vi "Dashboard Main_1920_1080.vi"() -> ()   [LabVIEW 2020]
uses:
  <vilib>/Rock Robotics/WPI/ThirdParty/JAS_Junk/TrajLib/TypeDef/FieldDisp_ElementPicture.ctl
  <vilib>/event_ctls.llb/eventvkey.ctl
  <vilib>/Rock Robotics/WPI/ThirdParty/JAS_Junk/TrajLib/Rotation2d_CreateAngle.vi
  <vilib>/Rock Robotics/WPI/ThirdParty/JAS_Junk/TrajLib/Translation2d_Create.vi
  <vilib>/Rock Robotics/WPI/ThirdParty/JAS_Junk/TrajLib/VI/FieldDisp_Element_Rotate.vi
  <vilib>/Rock Robotics/WPI/ThirdParty/JAS_Junk/TrajLib/Conv_Meters_Inches.vi
  <vilib>/Rock Robotics/WPI/ThirdParty/JAS_Junk/TrajLib/Conv_Radians_Deg.vi
  <vilib>/Rock Robotics/WPI/Dashboard/WPI_DashboardLogging Global.vi
  <vilib>/Rock Robotics/Network Tables/NT Read Numeric Array.vi
  <vilib>/picture/pixmap.llb/Flatten Pixmap.vi
  <vilib>/picture/pictutil.llb/Create Mask.vi
  <vilib>/picture/picture.llb/Draw Flattened Pixmap.vi
  <vilib>/Rock Robotics/WPI/ThirdParty/JAS_Junk/TrajLib/Trajectory_Library.lvlib
panel:
  out "Camera Perf":string
  in  "Camera Settings":T1={"Frame Rate"=30, "Compression"=30, "Size"=1, "DB Camera Config"=FALSE} {"Frame Rate" scale=1.0..30.0; "Compression" scale=100.0..-1.0; "Size" items=["640x480", "320x240", "160x120"]}
  in  "TCP":refnum<k5>
  in  "Rec Mode":enum32{"Stop", "Record", "Playback"}(radio)
  out "Robot IP":string
  out "Image Message":string="Timeout in Camera Communications"
  in  "Dashboard Tab":T2(tab)
  in  "Select Auto":string(combo)="Select Autonomous ..."
  out "NT Connection":bool
  out "MotorChart R":cluster{"Numeric":dbl, "Numeric":dbl}(graph)
  out "MotorChart L":cluster{"Numeric":dbl, "Numeric":dbl}(graph)
  out "MotorSliders R":cluster{"MotorSlide1":dbl, "MotorSlide2":dbl} {"MotorSlide2" scale=-1.0..1.0 scale format="%#_2e"; "MotorSlide1" scale=-1.0..1.0 scale format="%#_2e"}
  out "MotorSliders L":cluster{"MotorSlide1":dbl, "MotorSlide2":dbl} {"MotorSlide2" scale=-1.0..1.0 scale format="%#_2e"; "MotorSlide1" scale=-1.0..1.0 scale format="%#_2e"}
  out "Gyro":dbl(knob) scale=0.0..360.0
  out "JS1 Z":dbl(slide) scale=-1.0..1.0 scale format="%#_2e"
  out "JS1 Graph":cluster{"X":dbl, "Y":dbl}[](graph)
  out "JS1 Buttons":T3
  out "JS2 Z":dbl(slide) scale=-1.0..1.0 scale format="%#_2e"
  out "JS2 Graph":cluster{"X":dbl, "Y":dbl}[](graph)
  out "JS2 Buttons":T3
  out "Mode":T4(ring)=enum."Auto Disabled"
  out "Right Camera Perf":cluster{"Bandwidth (Mbps)":dbl, "FPS":dbl}
  in  "DB/String 9":string
  in  "DB/String 8":string
  in  "DB/String 7":string
  in  "DB/String 6":string
  in  "DB/String 5":string
  in  "DB/String 4":string
  in  "DB/String 3":string
  in  "DB/String 2":string
  in  "DB/String 1":string
  in  "DB/String 0":string
  in  "DB/Slider 0":dbl(slide) scale=0.0..5.0
  in  "DB/Slider 1":dbl(slide) scale=0.0..5.0
  in  "DB/Slider 2":dbl(slide) scale=0.0..5.0
  in  "DB/Slider 3":dbl(slide) scale=0.0..5.0
  out "DB/LED 3":bool
  out "DB/LED 2":bool
  out "DB/LED 1":bool
  out "DB/LED 0":bool
  in  "DB/Button 3":bool
  in  "DB/Button 2":bool
  in  "DB/Button 1":bool
  in  "DB/Button 0":bool caption="New Name"
  out "ROBOT":T5
  out "Field Picture":picture
  in  "Test Slider":dbl(slide) scale=0.0..100.0 scale format="%#_3g"
  in  "On/Off":bool caption="Solenoid"
  in  "Test Name":u16(ring) items=["Select the test to run..."]
  in  "Test Tree":string(tree)
  in  "Motor":cluster{"Value":dbl, "Enable":bool} {"Value" scale=-1.0..1.0 scale format="%#_3g"}
  out "Progress":T6 {"Test Progress" scale=0.0..100.0}
  in  "Rev/Fwd":cluster{"Forward":bool, "Reverse":bool}
  in  "Test Ring":u16(ring) items=["Monochrome", "Color"]
  in  "CheckList":i32(listbox)
  out "Tree":string(tree)
  out "Camera Image":T7(plugin-control)
  out "Background":bool
  in  "Camera Name":string(combo)="No Camera Selection"
  # "HW"
  # "Joysticks"
  # "Drive Motors"
  # "Front"
  # "Right"
  # "Left"
  # "Back"
  # "This tab is a great place for autonomous settings and robot-specific values.\nPlace controls and indicators inside this tab and match name to\nDashboard Variables on robot. You can also delete this comment."
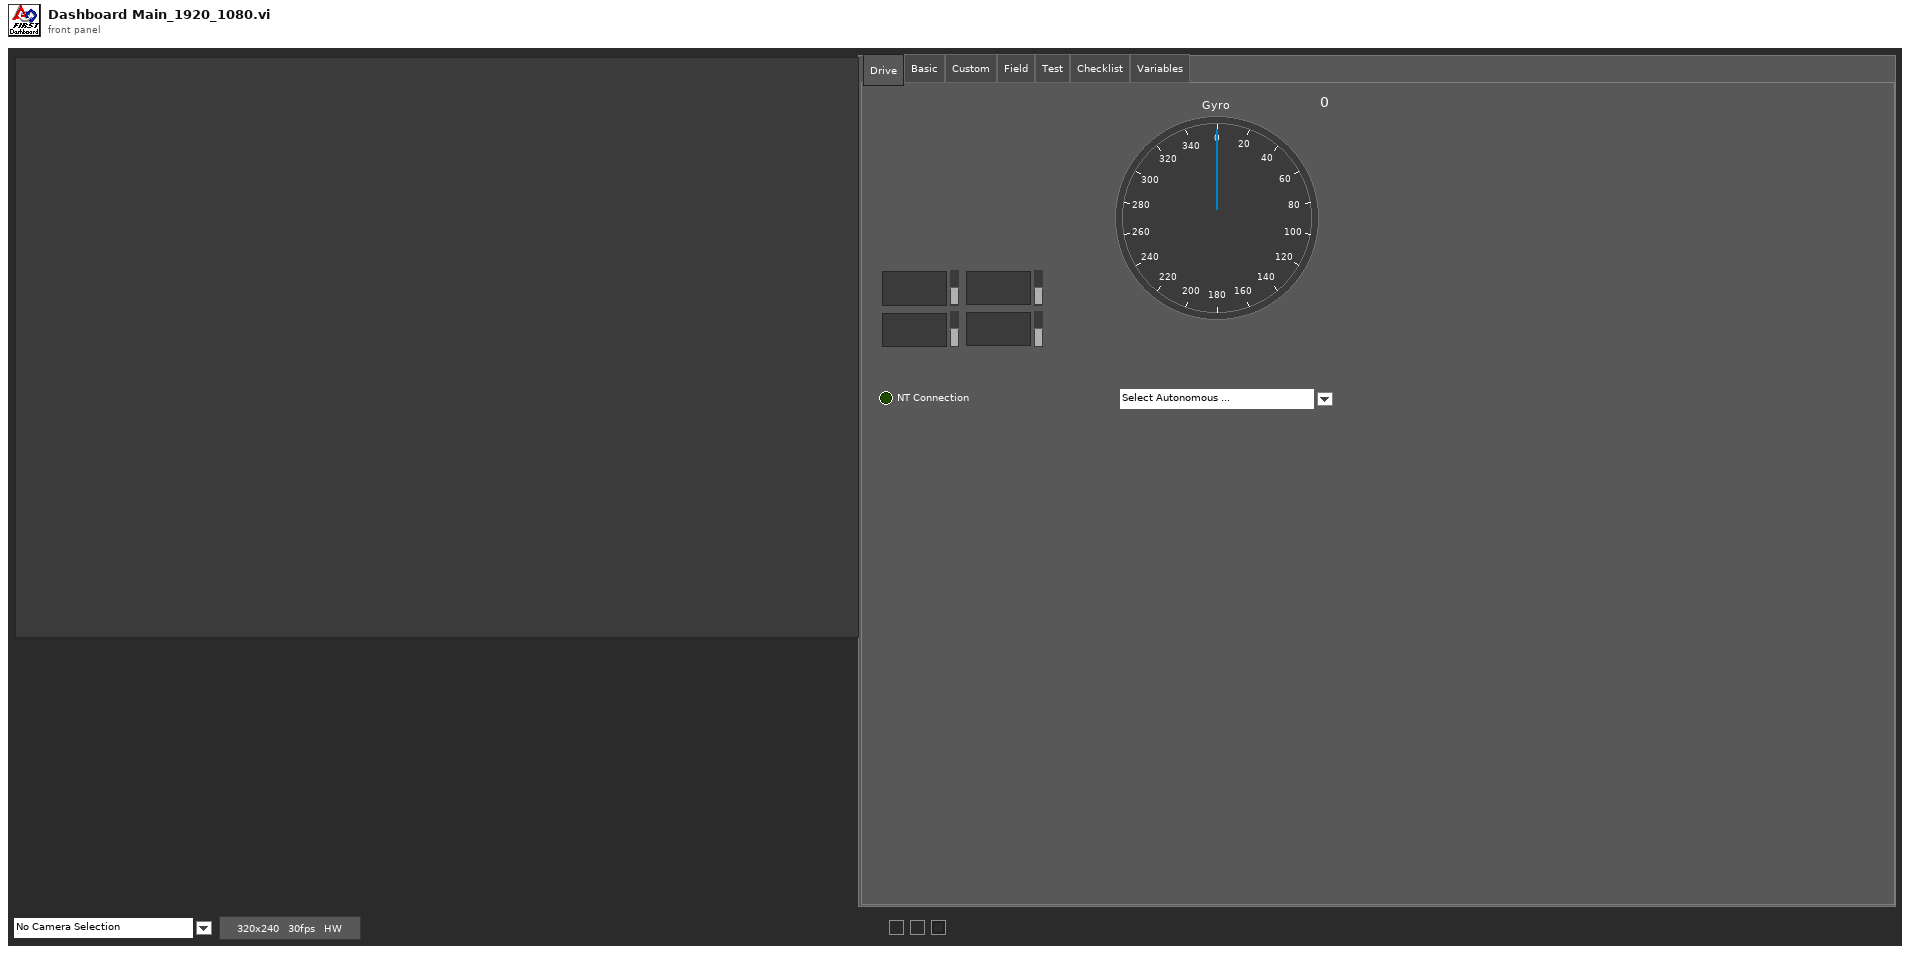
[diagram p1: front panel]
types:
  T1 = cluster{"Frame Rate":i32, "Compression":i32, "Size":u16, "DB Camera Config":bool}
  T2 = enum32{"Drive", "Basic", "Custom", "Field", "Test", "Checklist", "Variables"}
  T3 = cluster{bool, bool, bool, bool, bool, bool, bool, bool, bool, bool, bool, bool}
  T4 = enum8{"Tele-Op Disabled", "Tele-Op Enabled", "Auto Disabled", "Auto Enabled", "Test Disabled", "Test Enabled", "Disconnected", "No Code", "E-Stop"}
  T5 = typedef "Trajectory_Library.lvlib/FieldDisp_ElementPicture.ctl" = picture
  T6 = cluster{"Test Progress":u8, "Test Progress Text":string}
  T7 = typedef "IMAQ Image.ctl" = refnum<image>
  T8 = cluster{"Save Path":path, "Interval (s)":dbl, "Keep":i32}
  T9 = enum32{"Drive", "Camera", "Basic", "Custom", "Test", "Commands", "Checklist", "Variables"}
  T10 = typedef "Image Type" = u32
  T11 = cluster{"Camera Image":refnum<vi>, "Dashboard Tab":refnum<vi>, "Background":refnum<vi>, "Rec Mode":refnum<vi>, "Test Slider":refnum<vi>, "On/Off ":refnum<vi>, "Test Ring":refnum<vi>, "Rev/Fwd":refnum<vi>, "Test Name":refnum<vi>, "Motor":refnum<vi>, "Progress":refnum<vi>, "CheckList":refnum<vi>, "Tree":refnum<vi>, "Test Tree":refnum<vi>, "Camera Settings":refnum<vi>, "Camera Name":refnum<vi>, "Camera Perf":refnum<vi>}
  T12 = cluster{"Global Rectangle":i32[], "Contours":cluster{"Contour Type":u32, "ROI Type":u32, "Points":i32[]}[]}
  T13 = cluster{"Camera Name":string, string, "Saved DB Images Info":cluster{"Save Path":path, "Interval (s)":dbl, "Keep":i32}}
  T14 = cluster{"Operation":enum16{"Update", "Clear"}, "Color Box":u32}[]
  T15 = typedef "eventvkey.ctl" = enum16{"ASCII", "Enter", "Return", "Shift", "Ctrl", "Alt", "Cmd", "Opt", "Caps", "NumLock", "Clear", "Break", "Up", "Down", "Left", "Right", "Insert", "Delete", "Home", "End", "PageUp", "PageDown", "Escape", "Help", "Pause", "ScrollLock", "F1", "F2", "F3", "F4", "F5", "F6", "F7", "F8", "F9", "F10", "F11", "F12", "F13", "F14", "F15", "F16", "F17", "F18", "F19", "F20", "F21", "F22", "F23", "F24", "Play", "VolumeUp", "VolumeDown", "Mute", "Two Byte Char"}
  T16 = cluster{"Image Size":bool, "Image Type":bool, "Pixel Value":bool, "ROI Information":bool, "Zoom Factor":bool}
  T17 = cluster{"Operation":enum16{"Update", "Clear"}, "Color Box":u32}
  T18 = cluster{"Shift":bool, "Ctrl":bool, "Alt":bool, "Cmd":bool, "Opt":bool}
  T19 = typedef "Trajectory_Library.lvlib/FieldDisp_FieldElement.ctl" = cluster{"ONE-8-bit pixmap":u8[][], "Two-Array":cdb[][], "Three-Numeric":i32, "Four-Numeric":i32, "Five-Numeric":cdb, "Six-colors":u32[], "Seven-new element/subarray":u32, "Left Poxel":dbl, "Top Pixel":dbl, "Width Pix/Ft":dbl, "Height Pix/Ft":dbl, "Element Picture Ref":refnum<vi>}
  T20 = cluster{"Error Strings":string, "Disable Counts":cluster{u16, u16}, "Rail Faults":cluster{u16, u16, u16}, "Robot IP":string, "DB Mode":u8, "Event Info":cluster{"Name":string, "Type":u8, "Number":u16, "Replay":u8}}
  T21 = cluster{"Storage":cluster{"Disk Free":u64, "RAM Block":u32, "RAM free":u32}, "CPU Utilization":cluster{"CPU % ISR":sgl, "CPU % Time Crit":sgl, "CPU % Timed Str":sgl, "CPU % High":sgl, "CPU % Above":sgl, "CPU % Normal":sgl, "CPU % Low":sgl}, "CAN":cluster{"% Bus Utilization":sgl, "Bus Off Cnt":u32, "TX_FIFO Full Cnt":u32, "Receive Error Cnt":u8, "Transmit Error Cnt":u8}, "HID":cluster{"HID Outputs":u32, "Rumble Low":u16, "Rumble High":u16}[]}
  T22 = cluster{"Status bits":cluster{"Test Mode":bool, "Autonomous":bool, "Enabled":bool, "Code Start":bool, "Brownout":bool, "Reserved 2":bool, "Reserved 3":bool, "E-Stop":bool}, "Code Trace":cluster{"Disabled":bool, "TeleOp":bool, "Auto":bool, "Test":bool}, "Controller Type":enum16{"unknown", "cRIO", "roboRio"}, "Code?":enum16{"unknown", "noCode", "code"}, "Battery V":dbl}
  T23 = cluster{"Control Bits":cluster{"TestMode":bool, "Autonomous":bool, "Enabled":bool, "FMS Present":bool, bool, bool, bool, "E-Stop":bool}, "Team Station ":u8, "Countdown":sgl, "Joystick Values":cluster{"Axes":dbl[], "Buttons":bool[], "POVs":i16[]}[]}
  T24 = cluster{"Axes":dbl[], "Buttons":bool[], "POVs":i16[]}[]
  T25 = cluster{"Axes":dbl[], "Buttons":bool[], "POVs":i16[]}
  T26 = cluster{"Buttons[0]":bool, "Buttons[1]":bool, "Buttons[2]":bool, "Buttons[3]":bool, "Buttons[4]":bool, "Buttons[5]":bool, "Buttons[6]":bool, "Buttons[7]":bool, "Buttons[8]":bool, "Buttons[9]":bool, "Buttons[10]":bool, "Buttons[11]":bool}
  T27 = typedef "Trajectory_Library.lvlib/POSE2D.ctl" = cluster{"TRANSLATION":T28, "ROTATION":T29}
  T28 = typedef "Trajectory_Library.lvlib/TRANSLATION2D.ctl" = cluster{"X":dbl, "Y":dbl}
  T29 = typedef "Trajectory_Library.lvlib/ROTATION2D.ctl" = cluster{"VALUE":dbl, "COS":dbl, "SIN":dbl}
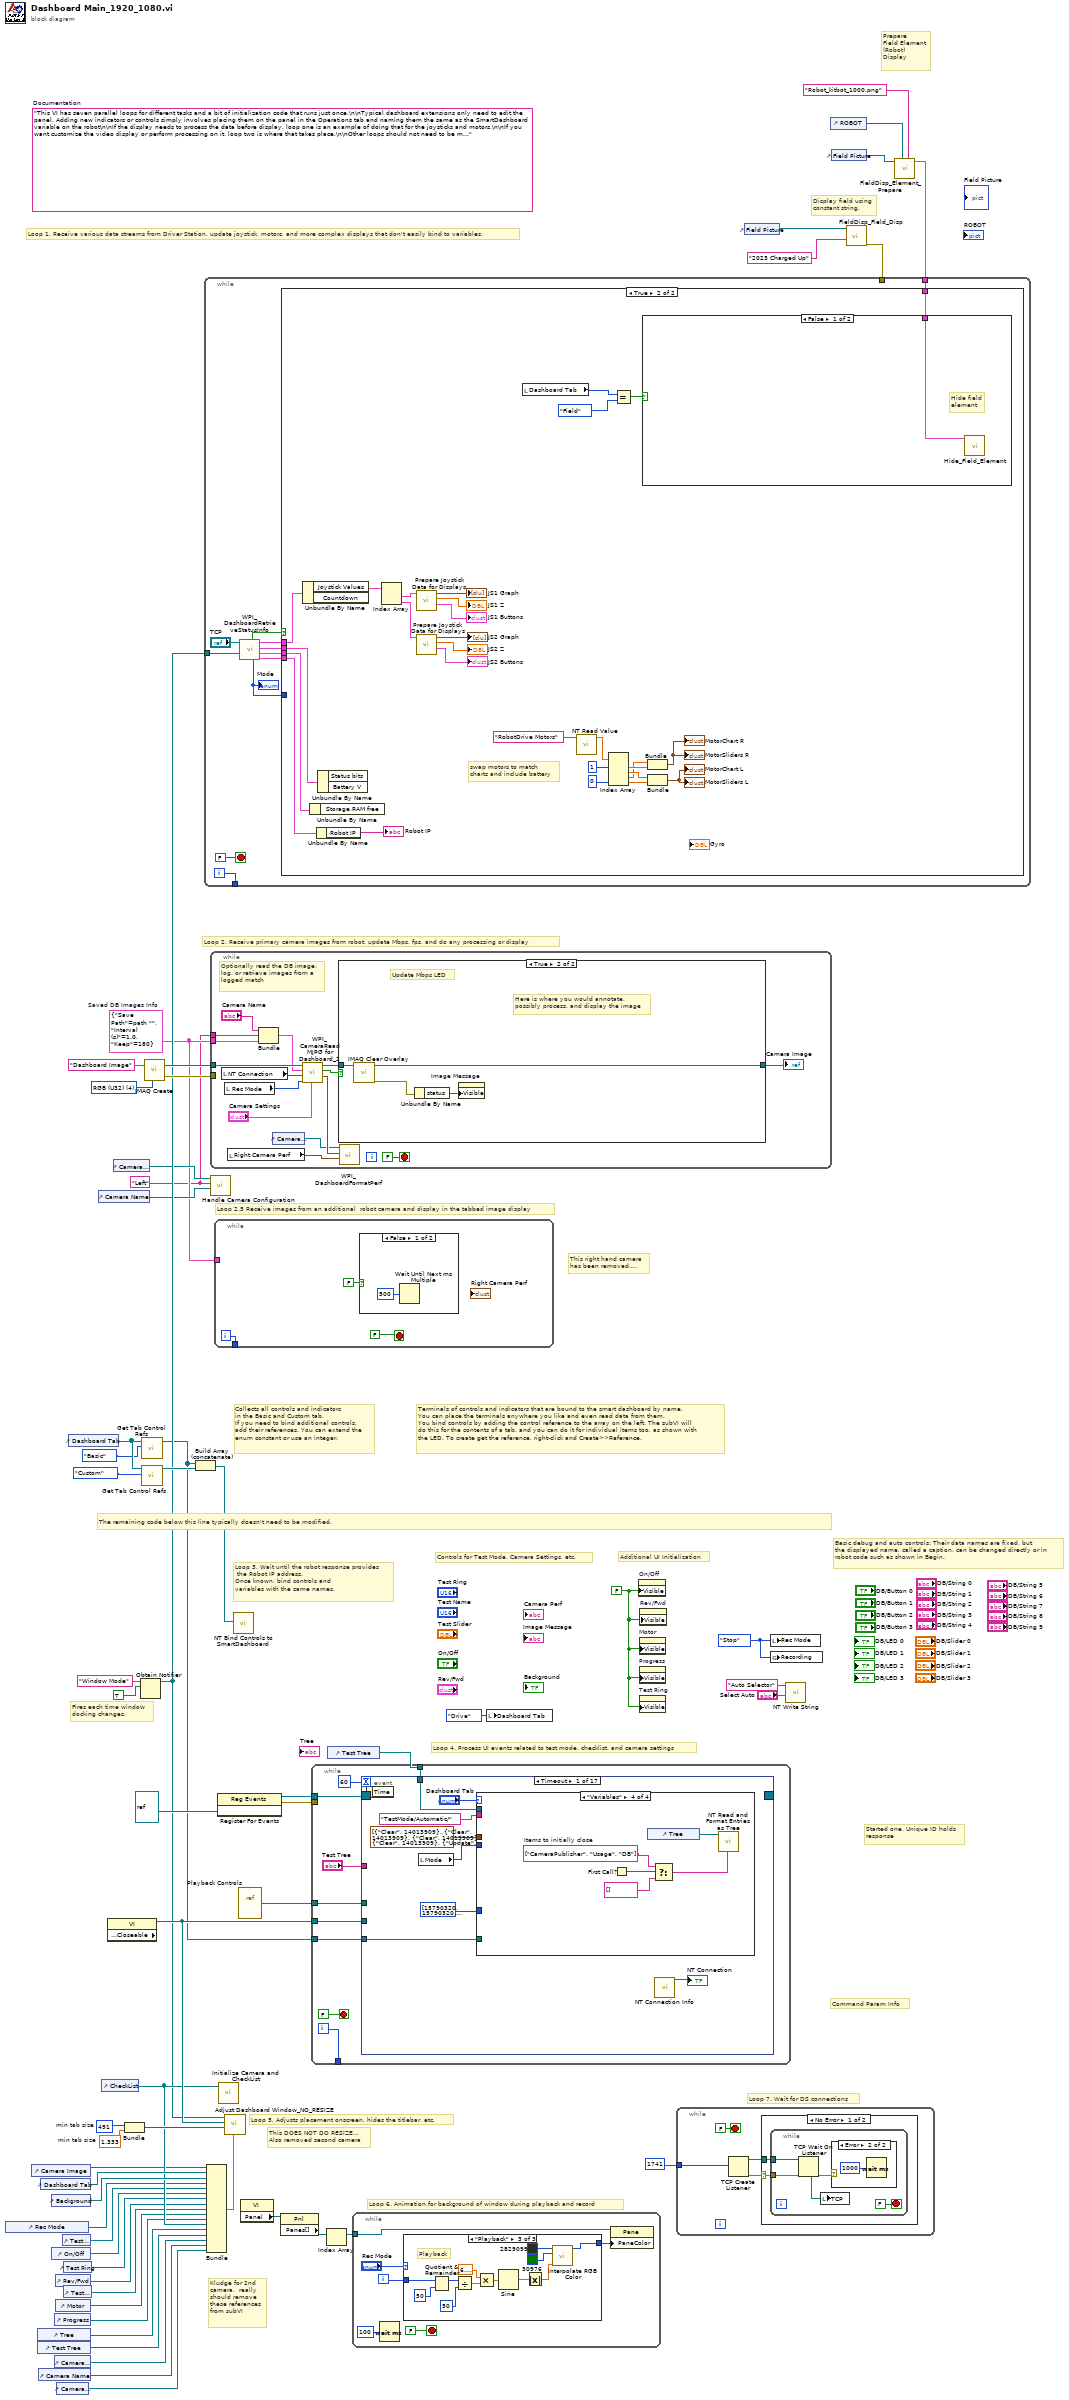
[diagram p0: block diagram]
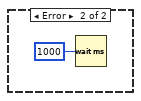
[diagram p4: hidden frame]
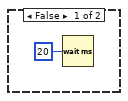
[diagram p5: hidden frame]
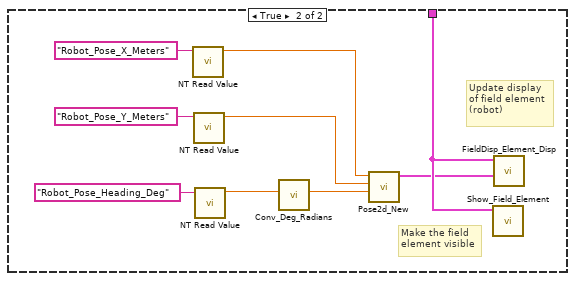
[diagram p6: hidden frame]
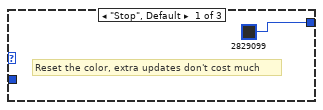
[diagram p7: hidden frame]
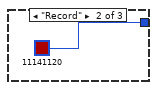
[diagram p8: hidden frame]
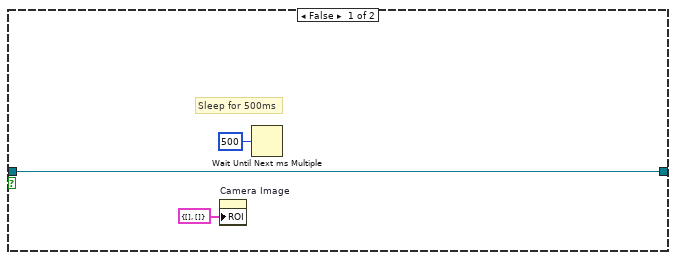
[diagram p9: hidden frame]
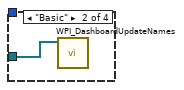
[diagram p11: hidden frame]
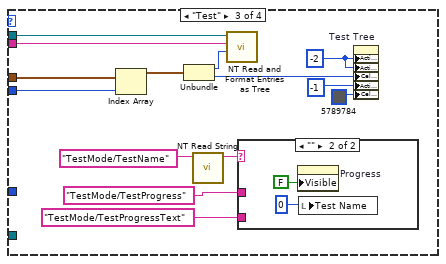
[diagram p12: hidden frame]
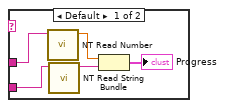
[diagram p13: hidden frame]
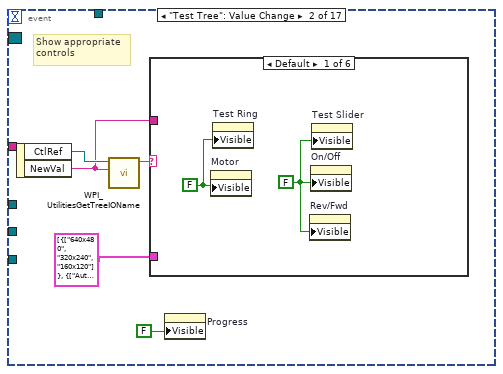
[diagram p14: hidden frame]
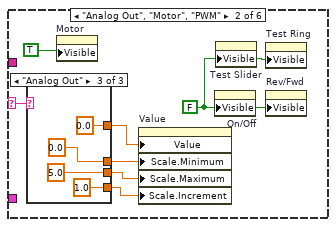
[diagram p15: hidden frame]
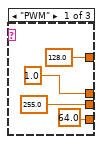
[diagram p16: hidden frame]
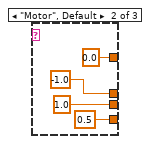
[diagram p17: hidden frame]
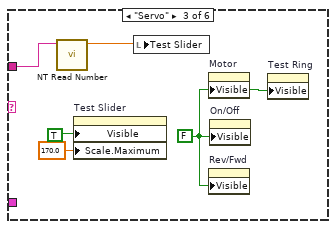
[diagram p18: hidden frame]
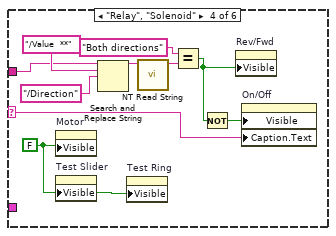
[diagram p19: hidden frame]
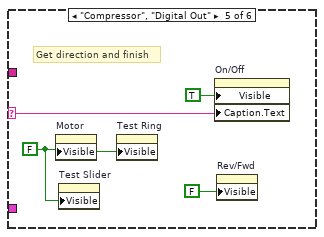
[diagram p20: hidden frame]
diagram:
  w13 = T8 {"Save Path"=path "", "Interval (s)"=1.0, "Keep"=180}  # Saved DB Images Info
  w12 = "Left"
  w40 = 491  # min tab size
  w39 = 1.333  # min tab size
  w46 = enum32{"Stop", "Record", "Playback"}."Stop" ("Rec Mode")
  w24 = FALSE ("Visible")
  (unwired) "This VI has seven parallel loops for different tasks and a bit of initialization code that runs just once.\n\nTypical dashboard extensions only need to edit the panel. Adding new indicators or controls simply involves placing them on the panel in the Operations tab and naming them the same as the SmartDashboard variable on the robot\n\nIf the display needs to process the data before display, loop one is an example of doing that for the joysticks and motors.\n\nIf you want customize the video display or perform processing on it, loop two is where that takes place.\n\nOther loops should not need to be modified. They are pretty standard, and document the task they perform."  # Documentation
  w60 = T10 4 items=["Grayscale (U8)", "Grayscale (I16)", "Grayscale (SGL)", "Complex (CSG)", "RGB (U32)", "HSL (U32)", "RGB (U64)"] ("Image Type")
  # "Display field using\nconstant string."
  # "Prepare\nField Element\n(Robot)\nDisplay"
  # "Kludge for 2nd\ncamera.  really\nshould remove\nthese references\nfrom subVI"
  # "This right hand camera\nhas been removed...."
  # "This DOES NOT DO RESIZE...\nAlso removed second camera"
  # "Loop 2.5 Receive images from an additional  robot camera and display in the tabbed image display"
  # "Command Param Info"
  # "Started one, Unique ID holds\nresponse"
  # "Loop 7. Wait for DS connections"
  # "Basic debug and auto controls: Their data names are fixed, but\nthe displayed name, called a caption, can be changed directly or in\nrobot code such as shown in Begin."
  # "Controls for Test Mode, Camera Settings, etc."
  # "Additional UI Initialization"
  # "Loop 6. Animation for background of window during playback and record"
  # "Fires each time window\ndocking changes."
  # "Collects all controls and indicators\nin the Basic and Custom tab.\nIf you need to bind additional controls,\nadd their references. You can extend the\nenum constant or use an integer."
  # "The remaining code below this line typically doesn't need to be modified."
  # "Loop 4. Process UI events related to test mode, checklist, and camera settings"
  # "Terminals of controls and indicators that are bound to the smart dashboard by name.\nYou can place the terminals anywhere you like and even read data from them.\nYou bind controls by adding the control reference to the array on the left. The subVI will\ndo this for the contents of a tab, and you can do it for individual items too, as shown with\nthe LED. To create get the reference, right-click and Create>>Reference."
  # "Loop 3. Wait until the robot response provides\n the Robot IP address.\nOnce known, bind controls and\nvariables with the same names."
  # "Loop 5. Adjusts placement onscreen, hides the titlebar, etc."
  # "Loop 1. Receive various data streams from Driver Station, update joystick, motors, and more complex displays that don't easily bind to variables."
  # "Loop 2. Receive primary camera images from robot, update Mbps, fps, and do any processing or display"
  n1 = control-ref of="Rec Mode"() -> (w30:refnum<vi>)
  n2 = control-ref of="Camera Image"() -> (w9:refnum<vi>)
  n3 = control-ref of="Tree"() -> (w34:refnum<vi>)
  n4 = control-ref of="Test Tree"() -> (w33:refnum<vi>)
  n5 = control-ref of="Camera Name"() -> (w10:refnum<vi>)
  n6 = control-ref of="Dashboard Tab"() -> (w41:refnum<vi>)
  n7 = control-ref of="Background"() -> (w37:refnum<vi>)
  n8 = control-ref of="On/Off"() -> (w28:refnum<vi>)
  n9 = control-ref of="Progress"() -> (w25:refnum<vi>)
  n10 = control-ref of="Camera Settings"() -> (w11:refnum<vi>)
  n11 = control-ref of="Rev/Fwd"() -> (w26:refnum<vi>)
  n12 = control-ref of="Motor"() -> (w31:refnum<vi>)
  n13 = control-ref of="Camera Perf"() -> (w19:refnum<vi>)
  n14 = control-ref of="Test Slider"() -> (w29:refnum<vi>)
  n15 = control-ref of="Test Ring"() -> (w27:refnum<vi>)
  n16 = control-ref of="Test Name"() -> (w32:refnum<vi>)
  n17 = control-ref of="Dashboard Tab"() -> (w44:refnum<vi>)
  n18 = control-ref of="Camera Name"() -> (w20:refnum<vi>)
  n19 = control-ref of="CheckList"() -> (w35:refnum<vi>)
  n20 = property class="VI" props=["Front Panel.Closeable"]() -> (reference out=w45:refnum<vi>)  [unwired: 2 in, 2 out]
  n21 = control-ref of="Camera Settings"() -> (w21:refnum<vi>)
  n22 = Bundle("min tab size"=w40, "min tab size"=w39) -> (w38:cluster{"min tab size":i32, "min tab size":dbl})  [unwired: 1 in]
  n23 = Obtain Notifier(name (unnamed)="Window Mode", notification data type=TRUE) -> (notifier out=w23:refnum<notifier>)  [unwired: 2 in, 2 out]
  n24 = call <vilib>:"Get Tab Control Refs.vi"("Page Index"=T9."Basic" ("Dashboard Tab"), "TabControl in"=w44) -> ("ControlsOnPage"=w18:refnum<vi>[])  [unwired: 9 in]
  n25 = call <vilib>:"Get Tab Control Refs.vi"("Page Index"=T9."Custom" ("Dashboard Tab"), "TabControl in"=w44) -> ("ControlsOnPage"=w43:refnum<vi>[])  [unwired: 9 in]
  n26 = call "IMAQ Create"("Image Name"="Dashboard Image", "Image Type"=w60) -> ("New Image"=w58:T7, "error out"=w57:errorcluster)  [unwired: 2 in, 1 out]
  n27 = Build Array (concatenate)(w18, w43) -> (w42:refnum<vi>[])
  n28 = Bundle("Camera Image"=w9, "Dashboard Tab"=w41, "Background"=w37, "Rec Mode"=w30, "Test Slider"=w29, "On/Off"=w28, "Test Ring"=w27, "Rev/Fwd"=w26, "Test Name"=w32, "Motor"=w31, "Progress"=w25, "CheckList"=w35, "Tree"=w34, "Test Tree"=w33, "Camera Settings"=w11, "Camera Name"=w10, "Camera Perf"=w19) -> (w36:T11)  [unwired: 1 in]
  n29 = call "Handle Camera Configuration.vi"("CameraNameRef"=w20, "Display Name"=w12, "ClusterRef"=w21) -> ()  [unwired: 9 in]
  n30 = while {
    tunnel: w58 -> [w74]
    tunnel: w57 -> [_]
    tunnel: w13 -> [w67]
    tunnel: w12 -> [w64]
    stop <- FALSE stop-if-true
    # "Optionally read the DB image,\nlog, or retrieve images from a\nlogged match"
    n31 = local read "NT Connection"() -> (w68:bool)
    n32 = local read "Rec Mode"() -> (w71:enum32{"Stop", "Record", "Playback"})
    n33 = local read "Right Camera Perf"() -> (w62:cluster{"Bandwidth (Mbps)":dbl, "FPS":dbl})
    n34 = Bundle("Camera Name"="Camera Name", w64, "Saved DB Images Info"=w67) -> (w66:T13)  [unwired: 1 in]
    n35 = control-ref of="Camera Perf"() -> (w61:refnum<vi>)
    n36 = call <vilib>:"WPI_CameraRead MJPG for Dashboard_2.vi"("Camera Settings"="Camera Settings", "Rec Mode"=w71, "NT Connection"=w68, "Capture Info"=w66, "Image in"=w74) -> ("perf info"=w63:cluster{"Bandwidth (Mbps)":dbl, "fps":dbl}, "Active"=w72:bool, "Image\\ out"=w73:T7)  [unwired: 4 in]
    n37 = case shown="True" w72 {
      tunnel: w73 -> [w77 w80]
      tunnel: [w77 w79] -> w69
      frame False {
        # "Sleep for 500ms"
        n38 = property on="Camera Image" class="ImageControl"("ROI"=T12 {"Global Rectangle"=[], "Contours"=[]}) -> ()  [unwired: 2 in, 2 out]
        n39 = Wait Until Next ms Multiple(millisecond multiple=u32 500) -> ()  [unwired: 1 out]
      }
      frame True {
        # "Here is where you would annotate,\npossibly process, and display the image"
        # "Update Mbps LED"
        n40 = call "IMAQ Clear Overlay"("Image"=w80) -> ("error out"=w81:errorcluster, "Image Out"=w79:T7)  [unwired: 2 in, 7 out]
        n41 = Unbundle By Name(w81) -> ("status"=w82:bool)
        n42 = property on="Image Message" class="Str"("Visible"=w82) -> ()  [unwired: 2 in, 2 out]
      }
    }
    "Camera Image" <- w69
    n43 = call <vilib>:"WPI_DashboardFormatPerf.vi"("Right Camera Perf"=w62, "Performance"=w63, "String in"=w61) -> ()  [unwired: 9 in]
  }
  n44 = while {
    tunnel: [w84] -> _
    tunnel: w13 -> [_]
    i -> [w84]
    stop <- FALSE stop-if-true
    n45 = case shown="False" FALSE {
      frame False {
        n46 = Wait Until Next ms Multiple(millisecond multiple=u32 500) -> ()  [unwired: 1 out]
      }
      frame True {
      }
    }
  }
  n47 = register-events(refnum<vi> refnum) -> (reference out=w49:refnum<event-registration>, error out=w48:errorcluster)  [unwired: 2 in]
  n48 = call "Initialize Camera and CheckList.vi"("ListBox in"=w35) -> ()  [unwired: 11 in]
  n49 = call "Adjust Dashboard Window_NO_RESIZE.vi"("Sizing Refnums"=w36, "Size Constraints"=w38, "VI"=w45, "WIn Mode"=w23) -> ()  [unwired: 8 in]
  n50 = call <vilib>:"NT Bind Controls to SmartDashboard.vi"("Bound Control Refs"=w42) -> ()  [unwired: 11 in]
  n51 = vi-ref "Playback Controls.vi"() -> (w50:refnum<vi>)
  n52 = property class="VI"() -> ("Panel"=w52:refnum<vi>)  [unwired: 2 in, 2 out]
  n53 = property class="Pnl"(reference=w52) -> ("Panes[]"=w53:refnum<vi>[])  [unwired: 1 in, 2 out]
  n54 = Index Array(array=w53) -> (element=w51:refnum<vi>)  [unwired: 1 in]
  n55 = control-ref of="Test Tree"() -> (w54:refnum<vi>)
  n56 = while {
    tunnel: [w92] -> _
    tunnel: w54 -> [w91]
    tunnel: w50 -> [w90]
    tunnel: w49 -> [w89]
    tunnel: w48 -> [_]
    tunnel: w45 -> [w88]
    tunnel: w18 -> [w87]
    i -> [w92]
    stop <- FALSE stop-if-true
    n57 = event shown="[0] Timeout" {
      selector: w89 -> [_ _ _ _ _ _ _ _ _ _ _ _ _ _ _ _ _]
      dyn-events: [_ _ _ _ _ _ _ _ _ _ _ _ _ w297 _ _ _] -> _
      timeout: u32 60 ("milliseconds to wait") -> [_ _ _ _ _ _ _ _ _ _ _ _ _ _ _ _ _]
      tunnel: w91 -> [w102 _ _ _ _ _ _ _ _ _ _ _ _ _ _ _ _]
      tunnel: "Test Tree" -> [_ _ _ _ _ _ _ _ w270 w277 w278 w281 w288 _ _ _ _]
      tunnel: w90 -> [_ _ _ _ _ _ _ _ _ _ _ _ _ w299 _ w314 _]
      tunnel: w88 -> [_ _ _ _ _ _ _ _ _ _ _ _ _ w295 _ _ _]
      tunnel: w87 -> [w97 _ _ _ _ _ _ _ _ _ _ _ _ _ _ _ _]
      event Timeout {
        n58 = event-data() -> ()  [unwired: 1 in, 1 out]
        n59 = local read "Mode"() -> (w100:T4)
        n60 = case shown="\"Variables\"" "Dashboard Tab" {
          tunnel: w102 -> [_ _ w118 _]
          tunnel: "TestMode/Automatic/" ("Name Pattern") -> [_ _ w117 _]
          tunnel: T14 [{"Operation"=enum."Clear", "Color Box"=14013909}, {"Operation"=enum."Clear", "Color Box"=14013909}, {"Operation"=enum."Clear", "Color Box"=14013909}, {"Operation"=enum."Clear", "Color Box"=14013909}, {"Operation"=enum."Update", "Color Box"=14013909}, {"Operation"=enum."Update", "Color Box"=16777215}, {"Operation"=enum."Clear", "Color Box"=14013909}, {"Operation"=enum."Clear", "Color Box"=14013909}, {"Operation"=enum."Clear", "Color Box"=14013909}] -> [_ _ w110 _]
          tunnel: w100 -> [_ _ w109 _]
          tunnel: u32[] [15790320, 15790320, 15790320, 15790320, 16777215, 16777215, 15790320, 15790320, 15790320] -> [_ _ _ _]
          tunnel: w97 -> [_ w104 _ _]
          frame "Custom", Default {
          }
          frame "Basic" {
            n61 = call <vilib>:"WPI_DashboardUpdateNames.vi"("Controls on Tab"=w104) -> ()  [unwired: 11 in]
          }
          frame "Test" {
            w116 = -2 ("Active Item:Row Number")
            n62 = Index Array(array=w110, index=w109) -> (element=w111:T17)
            n63 = Unbundle(w111) -> ("Operation"=w112:enum16{"Update", "Clear"}, "Color Box"=w113:u32)
            n64 = call <vilib>:"NT Read String.vi"("name"="TestMode/TestName" ("Name")) -> ("value"=w107:string)  [unwired: 8 in, 2 out]
            n65 = call <vilib>:"NT Read and Format Entries as Tree.vi"("Operation"=w112, "Name Pattern"=w117, "Tree Refnum"=w118) -> ()  [unwired: 7 in, 2 out]
            n66 = case shown="\"\"" w107 {
              tunnel: "TestMode/TestProgress" ("Name") -> [w120 _]
              tunnel: "TestMode/TestProgressText" ("Name") -> [w119 _]
              frame Default {
                n67 = call <vilib>:"NT Read Number.vi"("name"=w120) -> ("value"=w121:dbl)  [unwired: 8 in, 2 out]
                n68 = call <vilib>:"NT Read String.vi"("name"=w119) -> ("value"=w122:string)  [unwired: 8 in, 2 out]
                n69 = Bundle("value"=w121, "value"=w122) -> (→"Progress":cluster{"value":dbl, "value":string})  [unwired: 1 in]
              }
              frame "" {
                n70 = property on="Progress" class="Clust (strict)"("Visible"=FALSE) -> ()  [unwired: 2 in, 2 out]
                n71 = local write "Test Name"(u16 0) -> ()
              }
            }
            n72 = property on="Test Tree" class="Tree (strict)"("Active Item Row Number"=w116, "ActiveColNum"=w116, "CellBG"=w113, "Active Item Row Number"=-1 ("Active Item:Row Number"), "CellBG"=u32 5789784 ("Color Box")) -> ()  [unwired: 2 in, 2 out]
          }
          frame "Variables" {
            w128 = string[] ["CameraPublisher", "Usage", "DB"]  # Items to initially close
            n73 = First Call?() -> (First Call?: T/F=w129:bool)
            n74 = control-ref of="Tree"() -> (w130:refnum<vi>)
            n75 = Select(t=w128, s=w129, f=string[] []) -> (s? t:f=w126:string[])
            n76 = call <vilib>:"NT Read and Format Entries as Tree.vi"("Tags to  Close"=w126, "Tree Refnum"=w130) -> ()  [unwired: 8 in, 2 out]
          }
        }
        n77 = call <vilib>:"NT Connection Info.vi"() -> ("Connected"=→"NT Connection":bool)  [unwired: 11 in]
      }
      event "Test Tree": Value Change {
        # "Show appropriate\ncontrols"
        n78 = event-data() -> ("CtlRef"=w134:refnum<vi>, "NewVal"=w132:string)  [unwired: 1 in]
        n79 = call <vilib>:"WPI_UtilitiesGetTreeIOName.vi"("NewVal"=w132, "TreeControl in"=w134) -> ("I/O Name"=w135:string)  [unwired: 9 in]
        n80 = case shown="Default" w135 {
          selector: w135 -> [_ w142 _ w164 w173 _]
          tunnel: w132 -> [_ _ w161 w163 _ w180]
          tunnel: cluster{string[]}[] [{["640x480", "320x240", "160x120"]}, {["Auto", "Fixed indoor", "Fixed outdoor 1", "Fixed outdoor 2", "Fixed fluorescent 1", "Fixed fluorescent 2", "Hold current"]}, {["Auto", "Flicker-free 50 Hz", "Flicker-free 60 Hz", "Hold current"]}, {["None", "Prioritize frame rate", "Prioritize image quality"]}, {["Monochrome", "Color"]}] -> [_ _ _ _ _ w179]
          frame Default {
            w137 = FALSE ("Visible")
            w136 = FALSE ("Visible")
            n81 = property on="Motor" class="Clust (strict)"("Visible"=w136) -> ()  [unwired: 2 in, 2 out]
            n82 = property on="Test Ring" class="Ring (strict)"("Visible"=w136) -> ()  [unwired: 2 in, 2 out]
            n83 = property on="Rev/Fwd" class="Clust (strict)"("Visible"=w137) -> ()  [unwired: 2 in, 2 out]
            n84 = property on="On/Off" class="Bool (strict)"("Visible"=w137) -> ()  [unwired: 2 in, 2 out]
            n85 = property on="Test Slider" class="Slide (strict)"("Visible"=w137) -> ()  [unwired: 2 in, 2 out]
          }
          frame "Analog Out", "Motor", "PWM" {
            w143 = FALSE ("Visible")
            n86 = case shown="\"Analog Out\"" w142 {
              tunnel: [1.0 ("Value") -1.0 ("Value") 0.0 ("Value")] -> w141
              tunnel: [255.0 ("Value") 1.0 ("Value") 5.0 ("Value")] -> w140
              tunnel: [128.0 ("Value") 0.0 ("Value") 0.0 ("Value")] -> w139
              tunnel: [64.0 ("Value") 0.5 ("Value") 1.0 ("Value")] -> w138
              frame "PWM" {
              }
              frame "Motor", Default {
              }
              frame "Analog Out" {
              }
            }
            n87 = property on="Motor" class="Clust (strict)"("Visible"=TRUE) -> ()  [unwired: 2 in, 2 out]
            n88 = property on="Value" class="Slide (strict)"("Value"=w139, "Scale.Minimum"=w141, "Scale.Maximum"=w140, "Scale.Increment"=w138) -> ()  [unwired: 2 in, 2 out]
            n89 = property on="On/Off" class="Bool (strict)"("Visible"=w143) -> ()  [unwired: 2 in, 2 out]
            n90 = property on="Test Slider" class="Slide (strict)"("Visible"=w143) -> ()  [unwired: 2 in, 2 out]
            n91 = property on="Test Ring" class="Ring (strict)"("Visible"=w143) -> ()  [unwired: 2 in, 2 out]
            n92 = property on="Rev/Fwd" class="Clust (strict)"("Visible"=w143) -> ()  [unwired: 2 in, 2 out]
          }
          frame "Servo" {
            w159 = FALSE ("Visible")
            n93 = call <vilib>:"NT Read Number.vi"("name"=w161) -> ("value"=w160:dbl)  [unwired: 8 in, 2 out]
            n94 = property on="Test Slider" class="Slide (strict)"("Visible"=TRUE, "Scale.Maximum"=170.0 ("Scale.Range:Maximum")) -> ()  [unwired: 2 in, 2 out]
            n95 = local write "Test Slider"(w160) -> ()
            n96 = property on="Motor" class="Clust (strict)"("Visible"=w159) -> ()  [unwired: 2 in, 2 out]
            n97 = property on="Rev/Fwd" class="Clust (strict)"("Visible"=w159) -> ()  [unwired: 2 in, 2 out]
            n98 = property on="On/Off" class="Bool (strict)"("Visible"=w159) -> ()  [unwired: 2 in, 2 out]
            n99 = property on="Test Ring" class="Ring (strict)"("Visible"=w159) -> ()  [unwired: 2 in, 2 out]
          }
          frame "Relay", "Solenoid" {
            w162 = FALSE ("Visible")
            n100 = property on="Motor" class="Clust (strict)"("Visible"=w162) -> ()  [unwired: 2 in, 2 out]
            n101 = property on="Test Slider" class="Slide (strict)"("Visible"=w162) -> ()  [unwired: 2 in, 2 out]
            n102 = Search and Replace String(input string=w163, search string="/Value  **", replace string="/Direction") -> (result string=w169:string)  [unwired: 5 in, 3 out]
            n103 = property on="Test Ring" class="Ring (strict)"("Visible"=w162) -> ()  [unwired: 2 in, 2 out]
            n104 = call <vilib>:"NT Read String.vi"("name"=w169) -> ("value"=w167:string)  [unwired: 8 in, 2 out]
            n105 = Equal?(x="Both directions", y=w167) -> (x = y?=w165:bool)
            n106 = Not(x=w165) -> (.not. x?=w166:bool)
            n107 = property on="Rev/Fwd" class="Clust (strict)"("Visible"=w165) -> ()  [unwired: 2 in, 2 out]
            n108 = property on="On/Off" class="Bool (strict)"("Visible"=w166, "Caption.Text"=w164) -> ()  [unwired: 2 in, 2 out]
          }
          frame "Compressor", "Digital Out" {
            w172 = FALSE ("Visible")
            # "Get direction and finish"
            n109 = property on="Motor" class="Clust (strict)"("Visible"=w172) -> ()  [unwired: 2 in, 2 out]
            n110 = property on="Test Slider" class="Slide (strict)"("Visible"=w172) -> ()  [unwired: 2 in, 2 out]
            n111 = property on="Test Ring" class="Ring (strict)"("Visible"=w172) -> ()  [unwired: 2 in, 2 out]
            n112 = property on="On/Off" class="Bool (strict)"("Visible"=TRUE, "Caption.Text"=w173) -> ()  [unwired: 2 in, 2 out]
            n113 = property on="Rev/Fwd" class="Clust (strict)"("Visible"=FALSE) -> ()  [unwired: 2 in, 2 out]
          }
          frame "Camera" {
            n114 = call <vilib>:"NT_Get Last Path Segment.vi"("String in"=w180) -> ("String out"=w181:string)  [unwired: 10 in]
            n115 = property on="On/Off" class="Bool (strict)"("Visible"=FALSE) -> ()  [unwired: 2 in, 2 out]
            n116 = property on="Motor" class="Clust (strict)"("Visible"=FALSE) -> ()  [unwired: 2 in, 2 out]
            n117 = property on="Rev/Fwd" class="Clust (strict)"("Visible"=FALSE) -> ()  [unwired: 2 in, 2 out]
            n118 = case shown="\"White Balance  **\"" w181 {
              tunnel: w180 -> [w187 w196 w205 w214 w223 _ w229]
              tunnel: w179 -> [w185 w193 w202 w211 w220 _ _]
              frame "Size  **" {
                n119 = Index Array(array=w185) -> (element=w184:cluster{string[]})  [unwired: 1 in]
                n120 = call <vilib>:"NT Read String.vi"("name"=w187) -> ("value"=w186:string)  [unwired: 8 in, 2 out]
                n121 = Unbundle(w184) -> (w182:string[])
                n122 = Match First String(2:w182, 3:w186) -> (0:w183:i32)  [unwired: 1 out]
                n123 = property on="Test Ring" class="Ring (strict)"("Value"=w183, "Strings []"=w182) -> ()  [unwired: 2 in, 2 out]
                n124 = property on="Test Ring" class="Ring (strict)"("Visible"=TRUE) -> ()  [unwired: 2 in, 2 out]
                n125 = property on="Test Slider" class="Slide (strict)"("Visible"=FALSE) -> ()  [unwired: 2 in, 2 out]
              }
              frame "White Balance  **" {
                n126 = Index Array(array=w193, index=1) -> (element=w194:cluster{string[]})
                n127 = call <vilib>:"NT Read String.vi"("name"=w196) -> ("value"=w195:string)  [unwired: 8 in, 2 out]
                n128 = Unbundle(w194) -> (w191:string[])
                n129 = Match First String(2:w191, 3:w195) -> (0:w190:i32)  [unwired: 1 out]
                n130 = property on="Test Ring" class="Ring (strict)"("Value"=w190, "Strings []"=w191) -> ()  [unwired: 2 in, 2 out]
                n131 = property on="Test Ring" class="Ring (strict)"("Visible"=TRUE) -> ()  [unwired: 2 in, 2 out]
                n132 = property on="Test Slider" class="Slide (strict)"("Visible"=FALSE) -> ()  [unwired: 2 in, 2 out]
              }
              frame "Exposure  **" {
                n133 = Index Array(array=w202, index=2) -> (element=w203:cluster{string[]})
                n134 = call <vilib>:"NT Read String.vi"("name"=w205) -> ("value"=w204:string)  [unwired: 8 in, 2 out]
                n135 = Unbundle(w203) -> (w199:string[])
                n136 = Match First String(2:w199, 3:w204) -> (0:w200:i32)  [unwired: 1 out]
                n137 = property on="Test Ring" class="Ring (strict)"("Value"=w200, "Strings []"=w199) -> ()  [unwired: 2 in, 2 out]
                n138 = property on="Test Ring" class="Ring (strict)"("Visible"=TRUE) -> ()  [unwired: 2 in, 2 out]
                n139 = property on="Test Slider" class="Slide (strict)"("Visible"=FALSE) -> ()  [unwired: 2 in, 2 out]
              }
              frame "Exposure Priority  **" {
                n140 = Index Array(array=w211, index=3) -> (element=w212:cluster{string[]})
                n141 = call <vilib>:"NT Read String.vi"("name"=w214) -> ("value"=w213:string)  [unwired: 8 in, 2 out]
                n142 = Unbundle(w212) -> (w208:string[])
                n143 = Match First String(2:w208, 3:w213) -> (0:w209:i32)  [unwired: 1 out]
                n144 = property on="Test Ring" class="Ring (strict)"("Value"=w209, "Strings []"=w208) -> ()  [unwired: 2 in, 2 out]
                n145 = property on="Test Ring" class="Ring (strict)"("Visible"=TRUE) -> ()  [unwired: 2 in, 2 out]
                n146 = property on="Test Slider" class="Slide (strict)"("Visible"=FALSE) -> ()  [unwired: 2 in, 2 out]
              }
              frame "Color Enable  **" {
                n147 = Index Array(array=w220, index=4) -> (element=w221:cluster{string[]})
                n148 = call <vilib>:"NT Read String.vi"("name"=w223) -> ("value"=w222:string)  [unwired: 8 in, 2 out]
                n149 = Unbundle(w221) -> (w217:string[])
                n150 = Match First String(2:w217, 3:w222) -> (0:w218:i32)  [unwired: 1 out]
                n151 = property on="Test Ring" class="Ring (strict)"("Value"=w218, "Strings []"=w217) -> ()  [unwired: 2 in, 2 out]
                n152 = property on="Test Ring" class="Ring (strict)"("Visible"=TRUE) -> ()  [unwired: 2 in, 2 out]
                n153 = property on="Test Slider" class="Slide (strict)"("Visible"=FALSE) -> ()  [unwired: 2 in, 2 out]
              }
              frame Default {
                n154 = property on="Test Ring" class="Ring (strict)"("Visible"=FALSE) -> ()  [unwired: 2 in, 2 out]
                n155 = property on="Test Slider" class="Slide (strict)"("Visible"=FALSE) -> ()  [unwired: 2 in, 2 out]
              }
              frame "Brightness  **", "Color Level  **", "Compression  **", "FPS  **", "Sharpness  **" {
                n156 = call <vilib>:"NT Read Number.vi"("name"=w229) -> ("value"=w228:dbl)  [unwired: 8 in, 2 out]
                n157 = local write "Test Slider"(w228) -> ()
                n158 = property on="Test Slider" class="Slide (strict)"("Visible"=TRUE, "Scale.Maximum"=100.0 ("Scale.Range:Maximum")) -> ()  [unwired: 2 in, 2 out]
                n159 = property on="Test Ring" class="Ring (strict)"("Visible"=FALSE) -> ()  [unwired: 2 in, 2 out]
              }
            }
          }
        }
        n160 = property on="Progress" class="Clust (strict)"("Visible"=FALSE) -> ()  [unwired: 2 in, 2 out]
      }
      event "Test Name": Mouse Enter {
        # "Populate the ring with the list of tests"
        n161 = event-data() -> ()  [unwired: 1 in, 1 out]
        n162 = call <vilib>:"NT Read String Array.vi"("name"="TestMode/TestList" ("Name")) -> ("value"=w236:string[])  [unwired: 8 in, 2 out]
        n163 = Build Array (concatenate)("Select the test to run...", w236) -> (w235:string[])
        n164 = property on="Test Name" class="Ring (strict)"("Strings []"=w235) -> ()  [unwired: 2 in, 2 out]
      }
      event "Test Name": Value Change {
        w237 = FALSE ("Visible")
        # "Tell the robot the test name to run"
        n165 = event-data() -> ("NewVal"=w241:u16)  [unwired: 1 in]
        n166 = property on="Test Name" class="Ring (strict)"() -> ("Strings []"=w242:string[])  [unwired: 2 in, 2 out]
        n167 = local write "Progress"(T6 {"Test Progress"=0, "Test Progress Text"=""} ("Progress")) -> ()
        n168 = Index Array(array=w242, index=w241) -> (element=w240:string)
        n169 = call <vilib>:"NT Write String.vi"("value"=w240, "name"="TestMode/TestName" ("Name")) -> ()  [unwired: 9 in, 1 out]
        n170 = property on="Progress" class="Clust (strict)"("Visible"=TRUE) -> ()  [unwired: 2 in, 2 out]
        n171 = property on="Motor" class="Clust (strict)"("Visible"=w237) -> ()  [unwired: 2 in, 2 out]
        n172 = property on="Test Slider" class="Slide (strict)"("Visible"=w237) -> ()  [unwired: 2 in, 2 out]
        n173 = property on="On/Off" class="Bool (strict)"("Visible"=w237) -> ()  [unwired: 2 in, 2 out]
        n174 = property on="Rev/Fwd" class="Clust (strict)"("Visible"=w237) -> ()  [unwired: 2 in, 2 out]
        n175 = property on="Test Ring" class="Ring (strict)"("Visible"=w237) -> ()  [unwired: 2 in, 2 out]
      }
      event "Select Auto": Mouse Enter {
        # "Populate the combo box with the list of autonomous options"
        n176 = event-data() -> ()  [unwired: 1 in, 1 out]
        n177 = call <vilib>:"NT Read String Array.vi"("name"="Auto List" ("Name")) -> ("value"=w244:string[])  [unwired: 8 in, 2 out]
        n178 = property on="Select Auto" class="CmbBox"("Strings[]"=w244) -> ()  [unwired: 2 in, 2 out]
      }
      event "Select Auto": Value Change {
        # "User modified the Auto Selection. Write to NT variable so robot knows."
        n179 = event-data() -> ("NewVal"=w246:string)  [unwired: 1 in]
        n180 = call <vilib>:"NT Write String.vi"("value"=w246, "name"="Auto Selector" ("Name")) -> ()  [unwired: 9 in, 1 out]
      }
      event "CheckList": Double Click {
        # "Shift clears all"
        # "Update symbols on the listbox"
        n181 = event-data() -> ("PlatMods.Shift"=w248:bool, "Row"=w250:i32)  [unwired: 1 in]
        n182 = case shown="True" w248 {
          tunnel: w250 -> [w254 _]
          tunnel: 1 -> [w253 _]
          frame False {
            n183 = property on="CheckList" class="LstBox (strict)"() -> ("Item Symbols"=w252:i32[])  [unwired: 2 in, 2 out]
            n184 = Replace Array Subset(array=w252, new element=w253, index=w254) -> (w251:i32[])
            n185 = property on="CheckList" class="LstBox (strict)"("Item Symbols"=w251) -> ()  [unwired: 2 in, 2 out]
          }
          frame True {
            w255 = 0 ("Top Row")
            n186 = property on="CheckList" class="LstBox (strict)"() -> ("Number of Rows"=w257:u32)  [unwired: 2 in, 2 out]
            n187 = Initialize Array(0, w257) -> (w256:i32[])
            n188 = property on="CheckList" class="LstBox (strict)"("Top Row"=w255, "Value"=w255, "Item Symbols"=w256) -> ()  [unwired: 2 in, 2 out]
          }
        }
      }
      event "CheckList": Key Down {
        # "Update symbols on the listbox\nLeft and right keys check and uncheck"
        n189 = event-data() -> ("VKey"=w260:T15)  [unwired: 1 in]
        n190 = case shown="\"Left\", \"Right\"" w260 {
          selector: w260 -> [w265 _]
          tunnel: eventvkey."Left" ("VKey") -> [w263 _]
          frame "Left", "Right" {
            n191 = Equal?(x=w263, y=w265) -> (x = y?=w264:bool)
            n192 = Select(t=0, s=w264, f=1) -> (s? t:f=w266:i32)
            n193 = property on="CheckList" class="LstBox (strict)"() -> ("Item Symbols"=w269:i32[])  [unwired: 2 in, 2 out]
            n194 = Replace Array Subset(array=w269, new element=w266, index="CheckList") -> (w268:i32[])
            n195 = property on="CheckList" class="LstBox (strict)"("Item Symbols"=w268) -> ()  [unwired: 2 in, 2 out]
          }
          frame Default {
          }
        }
      }
      event "Motor.Enable": Value Change {
        # "When the test mode otor enable helper is set, update that\ntree row item's value"
        n196 = event-data() -> ("NewVal"=w274:bool)  [unwired: 1 in]
        n197 = Unbundle("Motor") -> ("Value"=w273:dbl)  [unwired: 1 out]
        n198 = Select(t=w273, s=w274, f=0.0) -> (s? t:f=w271:dbl)
        n199 = call <vilib>:"NT Write Number.vi"("value"=w271, "name"=w270) -> ()  [unwired: 9 in, 1 out]
      }
      event "Test Slider": Value Change {
        # "When the test mode slider helper is set, update that\ntree row item's value"
        n200 = event-data() -> ("NewVal"=w276:dbl)  [unwired: 1 in]
        n201 = call <vilib>:"NT Write Number.vi"("value"=w276, "name"=w277) -> ()  [unwired: 9 in, 1 out]
      }
      event "On/Off": Value Change {
        # "When the test mode on/off helper value is set, update that\ntree row item's value"
        n202 = event-data() -> ("NewVal"=w280:bool)  [unwired: 1 in]
        n203 = Boolean To (0,1)(Boolean=w280) -> (0, 1=w279:i16)
        n204 = call <vilib>:"NT Write Number.vi"("value"=w279, "name"=w278) -> ()  [unwired: 9 in, 1 out]
      }
      event "Rev/Fwd": Value Change {
        # "When the test mode helper value for relays is set, update that\ntree row item's value"
        n205 = event-data() -> ("NewVal.Forward"=w287:bool, "NewVal.Reverse"=w286:bool)  [unwired: 1 in]
        n206 = Boolean To (0,1)(Boolean=w287) -> (0, 1=w283:i16)
        n207 = Boolean To (0,1)(Boolean=w286) -> (0, 1=w285:i16)
        n208 = Negate(x=w285) -> (-x=w284:i16)
        n209 = Add(x=w283, y=w284) -> (x+y=w282:i16)
        n210 = call <vilib>:"NT Write Number.vi"("value"=w282, "name"=w281) -> ()  [unwired: 9 in, 1 out]
      }
      event "Test Ring": Value Change {
        # "When a test mode helper value is selected from the ring,\nset the tree item's variable to the string value"
        n211 = event-data() -> ("NewVal"=w290:u16)  [unwired: 1 in]
        n212 = property on="Test Ring" class="Ring (strict)"() -> ("Strings []"=w291:string[])  [unwired: 2 in, 2 out]
        n213 = Index Array(array=w291, index=w290) -> (element=w289:string)
        n214 = call <vilib>:"NT Write String.vi"("value"=w289, "name"=w288) -> ()  [unwired: 9 in, 1 out]
      }
      event "Rec Mode": Value Change {
        # "Update globals for recording mode and path to read log from.\nClear when logging and let NetworkTables set path for vision to\nuse."
        n215 = event-data() -> ("NewVal"=w300:enum32{"Stop", "Record", "Playback"})  [unwired: 1 in]
        n216 = global write "WPI_DashboardLogging Global.vi" "Logging Filename"(path "") -> ()
        n217 = global write "WPI_DashboardLogging Global.vi" "Recording"(w300) -> ()
        n218 = case shown="\"Playback\"" w300 {
          tunnel: w299 -> [_ w302 w310]
          tunnel: [_ _ w309] -> w297
          tunnel: [_ _ w308] -> _
          tunnel: w295 -> [_ _ w306]
          tunnel: cluster{i32, i32} {-250, 170} -> [_ _ w305]
          tunnel: [_ _ T16 {"Image Size"=TRUE, "Image Type"=TRUE, "Pixel Value"=TRUE, "ROI Information"=TRUE, "Zoom Factor"=FALSE} ("Image Information Shown:All Elements")] -> w292
          tunnel: [_ _ TRUE ("Zoom Factor")] -> w293
          frame Default {
          }
          frame "Stop", "Record" {
            # "Place Window too"
            n219 = invoke class="VI" method="FP.Close"(reference=w302) -> (reference out=w301:refnum<vi>)  [unwired: 2 in, 2 out]
            n220 = invoke class="VI" method="Abort VI"(reference=w301) -> ()  [unwired: 2 in, 3 out]
          }
          frame "Playback" {
            n221 = call "Open Playback Panel.vi"("Offset"=w305, "DB VI Ref"=w306, "Playback in"=w310) -> ("Playback out"=w307:refnum<vi>)  [unwired: 8 in]
            n222 = register-events(w307) -> (reference out=w309:refnum<event-registration>, error out=w308:errorcluster)  [unwired: 2 in]
          }
        }
        n223 = property on="Camera Image" class="ImageControl"("Image Information Shown"=w292, "Image Information Visible"=w293) -> ()  [unwired: 2 in, 2 out]
        n224 = call <vilib>:"WPI_DashboardNT Log FieldName Cache.vi"("Operation"=enum16{"Lookup/Add", "Index", "Clear"}."Clear") -> ()  [unwired: 8 in, 3 out]
      }
      event Panel Close {
        w311 = enum32{"Stop", "Record", "Playback"}."Stop" ("Rec Mode")
        # "Playback window has been closed, abort"
        n225 = event-data() -> ()  [unwired: 1 in, 4 out]
        n226 = local write "Rec Mode"(w311) -> ()
        n227 = global write "WPI_DashboardLogging Global.vi" "Recording"(w311) -> ()
      }
      event Panel Close {
        # "Abort playback window and ourself"
        n228 = event-data() -> ()  [unwired: 1 in, 4 out]
        n229 = invoke class="VI" method="FP.Close"(reference=w314) -> (reference out=w313:refnum<vi>)  [unwired: 2 in, 2 out]
        n230 = invoke class="VI" method="Abort VI"(reference=w313) -> (error out=w312:errorcluster)  [unwired: 2 in, 2 out]
        n231 = invoke class="VI" method="Abort VI"(error in=w312) -> ()  [unwired: 2 in, 3 out]
      }
      event "Tree": Double Click {
        n232 = event-data() -> ("PlatMods"=w320:T18, "Tag"=w317:string)  [unwired: 1 in]
        n233 = Unbundle(w320) -> ("Shift"=w319:bool)  [unwired: 4 out]
        n234 = String Subset(string=w317, length (rest)=1 ("length (rest)")) -> (substring=w316:string)  [unwired: 1 in]
        n235 = Not(x=w319) -> (.not. x?=w318:bool)
        n236 = case shown="\"/\"" w316 {
          tunnel: w317 -> [_ w322]
          tunnel: w318 -> [_ w321]
          frame Default {
          }
          frame "/" {
            n237 = call <vilib>:"NT Update Persistence.vi"("Persistence"=w321, "Name"=w322) -> ()  [unwired: 9 in, 1 out]
          }
        }
      }
    }
  }
  n238 = while {
    tunnel: w51 -> [w324]
    i -> [w327]
    stop <- FALSE stop-if-true
    n239 = Wait (ms)(milliseconds to wait=u32 100) -> ()  [unwired: 1 out]
    n240 = case shown="\"Playback\"" "Rec Mode" {
      tunnel: w327 -> [_ _ w342]
      tunnel: [u32 2829099 ("Base Color") u32 11141120 ("Target Color") w331] -> w323
      frame "Stop", Default {
        # "Reset the color, extra updates don't cost much"
      }
      frame "Record" {
      }
      frame "Playback" {
        # "Playback"
        n241 = Quotient & Remainder(x=w342, y=u32 50 ("milliseconds to wait")) -> (x-y*floor(x/y)=w338:u32)  [unwired: 1 out]
        n242 = Divide(x=w338, y=u32 50 ("milliseconds to wait")) -> (x/y=w335:dbl)
        n243 = Multiply(x=6.283185307179586, y=w335) -> (x*y=w340:dbl)
        n244 = Sine(x=w340) -> (sin(x)=w339:dbl)
        n245 = Absolute Value(x=w339) -> (abs(x)=w332:dbl)
        n246 = call "Interpolate RGB Color.vi"("Proportion"=w332, "Target Color"=u32 30976, "Base Color"=u32 2829099) -> ("Result Color"=w331:u32)  [unwired: 8 in]
      }
    }
    n247 = property class="Pane"(reference=w324, "PaneColor"=w323) -> ()  [unwired: 1 in, 2 out]
  }
  n248 = local write "Dashboard Tab"(T2."Drive" ("Dashboard Tab")) -> ()
  n249 = property on="On/Off" class="Bool (strict)"("Visible"=w24) -> ()  [unwired: 2 in, 2 out]
  n250 = property on="Motor" class="Clust (strict)"("Visible"=w24) -> ()  [unwired: 2 in, 2 out]
  n251 = property on="Progress" class="Clust (strict)"("Visible"=w24) -> ()  [unwired: 2 in, 2 out]
  n252 = property on="Test Ring" class="Ring (strict)"("Visible"=w24) -> ()  [unwired: 2 in, 2 out]
  n253 = property on="Rev/Fwd" class="Clust (strict)"("Visible"=w24) -> ()  [unwired: 2 in, 2 out]
  n254 = while {
    tunnel: u16 1741 ("timeout ms (25000)") -> [w344]
    stop <- FALSE stop-if-true
    n255 = TCP Create Listener(10:w344) -> (0:w343:errorcluster, 3:w345:refnum<k5>)  [unwired: 4 in, 1 out]
    n256 = case shown="No Error" w343 {
      selector: w343 -> [w347 _]
      tunnel: w345 -> [w348 _]
      frame No Error {
        n257 = while {
          tunnel: w348 -> [w351]
          tunnel: w347 -> [w350]
          stop <- FALSE stop-if-true
          n258 = TCP Wait On Listener(8:w350, 11:w351) -> (0:w352:errorcluster, 4:w353:refnum<k5>)  [unwired: 2 in, 3 out]
          n259 = local write "TCP"(w353) -> ()
          n260 = case shown="Error" w352 {
            frame No Error {
            }
            frame Error {
              n261 = Wait (ms)(milliseconds to wait=u32 1000) -> ()  [unwired: 1 out]
            }
          }
        }
      }
      frame Error {
        n262 = Wait (ms)(milliseconds to wait=u32 1000) -> ()  [unwired: 1 out]
      }
    }
  }
  n263 = control-ref of="Field Picture"() -> (w5:refnum<vi>)
  n264 = global write "WPI_DashboardLogging Global.vi" "Recording"(w46) -> ()
  n265 = local write "Rec Mode"(w46) -> ()
  n266 = call <vilib>:"NT Write String.vi"("value"="Select Auto", "name"="Auto Selector" ("Name")) -> ()  [unwired: 9 in, 1 out]
  n267 = control-ref of="ROBOT"() -> (w7:refnum<vi>)
  n268 = control-ref of="Field Picture"() -> (w8:refnum<vi>)
  n269 = call <vilib>:"FieldDisp_Field_Disp.vi"("Field Selector"="2023 Charged Up", "Picture in"=w5) -> ("error out"=w3:errorcluster)  [unwired: 9 in]
  n270 = call <vilib>:"FieldDisp_Element_Prepare.vi"("Element File Name"="Robot_kitbot_1000.png" ("Picture FIle Name"), "Element Picture Ref"=w7, "Field Picture Ref"=w8) -> ("Field Element Info"=w2:T19)  [unwired: 7 in, 1 out]
  n271 = while {
    tunnel: [w365] -> _
    tunnel: w23 -> [w357]
    tunnel: w3 -> [_]
    tunnel: w2 -> [w356]
    i -> [w365]
    stop <- FALSE stop-if-true
    n272 = call <vilib>:"WPI_DashboardRetrieveStatusInfo.vi"("Window Mode Notifier"=w357, "TCP Cnx"="TCP") -> ("Power and Errors"=w360:T20, "Robot Metrics"=w363:T21, "Status Info"=w364:T22, "Control Info"=w361:T23, "Robot Mode"=w359:T4, "Process?"=w362:bool)  [unwired: 4 in]
    "Mode" <- w359
    n273 = case shown="True" w362 {
      tunnel: w364 -> [_ w395]
      tunnel: w363 -> [_ w394]
      tunnel: w361 -> [_ w393]
      tunnel: w360 -> [_ w392]
      tunnel: w359 -> [_ _]
      tunnel: w356 -> [_ w371]
      frame False {
        n274 = Wait (ms)(milliseconds to wait=u32 20) -> ()  [unwired: 1 out]
      }
      frame True {
        # "swap motors to match\ncharts and include battery"
        n275 = Unbundle By Name(w393) -> ("Joystick Values"=w383:T24)  [unwired: 1 out]
        n276 = Unbundle By Name(w394) -> ()  [unwired: 1 out]
        n277 = Unbundle By Name(w392) -> ("Robot IP"=→"Robot IP":string)
        n278 = Unbundle By Name(w395) -> ()  [unwired: 2 out]
        n279 = Index Array(array=w383) -> (element #1=w382:T25, element #2=w378:T25)  [unwired: 2 in]
        n280 = call "Prepare Joystick Data for Displays.vi"("Joystick Values"=w378) -> ("Buttons"=→"JS2 Buttons":T26, "Z Axis"=→"JS2 Z":dbl, "Cartesian Data"=→"JS2 Graph":cluster{"X axis":dbl, "X axis":dbl}[])  [unwired: 8 in]
        n281 = call "Prepare Joystick Data for Displays.vi"("Joystick Values"=w382) -> ("Buttons"=→"JS1 Buttons":T26, "Z Axis"=→"JS1 Z":dbl, "Cartesian Data"=→"JS1 Graph":cluster{"X axis":dbl, "X axis":dbl}[])  [unwired: 8 in]
        n282 = local read "Dashboard Tab"() -> (w368:T2)
        n283 = call-poly <vilib>:"NT Read Value.vi"("name"="RobotDrive Motors" ("Name")) -> ("value"=w373:dbl[])  [unwired: 8 in, 2 out]
        n284 = Index Array(array=w373, index #1=1, index #4=0) -> (element #1=w387:dbl, element #2=w388:dbl, element #3=w386:dbl, element #4=w391:dbl)  [unwired: 2 in]
        n285 = Equal?(x=w368, y=T2."Field" ("Dashboard Tab")) -> (x = y?=w370:bool)
        n286 = case shown="False" w370 {
          tunnel: w371 -> [w396 w405]
          frame False {
            # "Hide field\nelement"
            n287 = call "Hide_Field_Element.vi"("Field Element Info"=w396) -> ()  [unwired: 11 in]
          }
          frame True {
            # "Make the field\nelement visible"
            # "Update display\nof field element\n(robot)"
            n288 = call-poly <vilib>:"NT Read Value.vi"("name"="Robot_Pose_X_Meters") -> ("value"=w398:dbl)  [unwired: 8 in, 2 out]
            n289 = call-poly <vilib>:"NT Read Value.vi"("name"="Robot_Pose_Y_Meters") -> ("value"=w397:dbl)  [unwired: 8 in, 2 out]
            n290 = call-poly <vilib>:"NT Read Value.vi"("name"="Robot_Pose_Heading_Deg") -> ("value"=w399:dbl)  [unwired: 8 in, 2 out]
            n291 = call <vilib>:"Conv_Deg_Radians.vi"("Degress"=w399) -> ("Radians"=w401:dbl)  [unwired: 10 in]
            n292 = call <vilib>:"Pose2d_New.vi"("Heading"=w401, "Y"=w397, "X"=w398) -> ("out POSe"=w400:T27)  [unwired: 8 in]
            n293 = call "Show_Field_Element.vi"("Field Element Info"=w405) -> ()  [unwired: 11 in]
            n294 = call <vilib>:"FieldDisp_Element_Disp.vi"("Element Pose"=w400, "Element Info"=w405) -> ()  [unwired: 10 in]
          }
        }
        n295 = Bundle("Numeric"=w386, "Numeric"=w387) -> (→"MotorChart R" →"MotorSliders R":cluster{"Numeric":dbl, "Numeric":dbl})  [unwired: 1 in]
        n296 = Bundle("Numeric"=w388, "Numeric"=w391) -> (→"MotorChart L" →"MotorSliders L":cluster{"Numeric":dbl, "Numeric":dbl})  [unwired: 1 in]
      }
    }
  }
